vi "Set Button Positions.vi"(6 "Top":i32, 8 "error in":errorcluster, 9 "List Right":i16, 10 "label array in":string[](array[string]), 11 "controls[] in":refnum<vi>[](array[refnum])) -> (0 "error out":errorcluster)   [LabVIEW 2018]
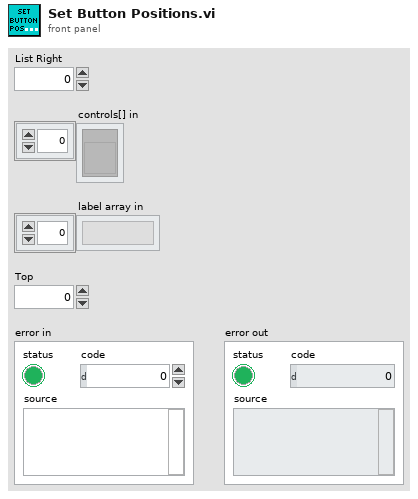
[diagram p1: front panel]
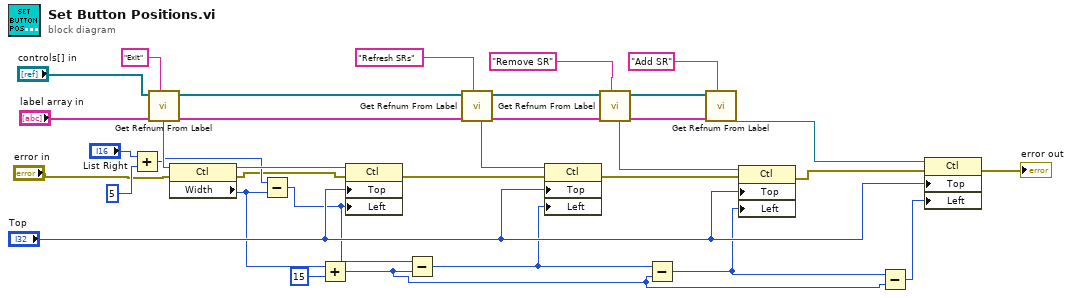
[diagram p0: block diagram]
diagram:
  n1 = Add(x="List Right", y=5) -> (x+y=w9:i32)
  n2 = call "Get Refnum From Label.vi"("label"="Exit" ("element"), "label array in"="label array in", "controls[] in"="controls[] in") -> ("label array out"=w25:string[], "controls[] out"=w26:refnum<vi>[], "refnum out"=w13:refnum<vi>)  [unwired: 6 in]
  n3 = property class="Ctl"(reference=w13, error in="error in") -> (reference out=w12:refnum<vi>, error out=w8:errorcluster, "Width"=w6:u32)
  n4 = Subtract(x=w9, y=w6) -> (x-y=w5:u32)
  n5 = Add(x=w6, y=i16 15) -> (x+y=w1:u32)
  n6 = property class="Ctl"(reference=w12, error in=w8, "Top"="Top", "Left"=w5) -> (error out=w22:errorcluster)  [unwired: 1 out]
  n7 = Subtract(x=w5, y=w1) -> (x-y=w4:u32)
  n8 = call "Get Refnum From Label.vi"("label"="Refresh SRs" ("element"), "label array in"=w25, "controls[] in"=w26) -> ("label array out"=w24:string[], "controls[] out"=w23:refnum<vi>[], "refnum out"=w18:refnum<vi>)  [unwired: 6 in]
  n9 = property class="Ctl"(reference=w18, error in=w22, "Top"="Top", "Left"=w4) -> (error out=w20:errorcluster)  [unwired: 1 out]
  n10 = call "Get Refnum From Label.vi"("label"="Remove SR" ("element"), "label array in"=w24, "controls[] in"=w23) -> ("label array out"=w33:string[], "controls[] out"=w34:refnum<vi>[], "refnum out"=w32:refnum<vi>)  [unwired: 6 in]
  n11 = Subtract(x=w4, y=w1) -> (x-y=w2:u32)
  n12 = call "Get Refnum From Label.vi"("label"="Add SR" ("element"), "label array in"=w33, "controls[] in"=w34) -> ("refnum out"=w31:refnum<vi>)  [unwired: 6 in, 2 out]
  n13 = property class="Ctl"(reference=w32, error in=w20, "Top"="Top", "Left"=w2) -> (error out=w19:errorcluster)  [unwired: 1 out]
  n14 = Subtract(x=w2, y=w1) -> (x-y=w3:u32)
  n15 = property class="Ctl"(reference=w31, error in=w19, "Top"="Top", "Left"=w3) -> (error out=→"error out":errorcluster)  [unwired: 1 out]
